vi "simple_tsv_recording.vi"(7 "file_base_name":string="simple_record", 8 "value":dbl format="%#_13g", 11 "date_time":timestamp) -> ()   [LabVIEW 2019]
uses:
  <vilib>/Utility/file.llb/Write Delimited Spreadsheet (string).vi
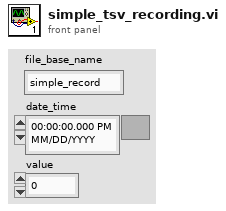
[diagram p1: front panel]
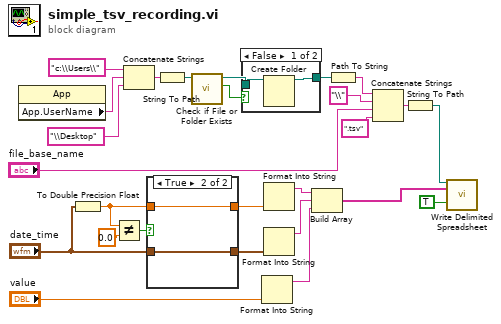
[diagram p0: block diagram]
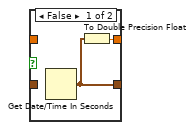
[diagram p2: hidden frame]
diagram:
  n1 = property class="App"() -> ("App.UserName"=w23:string)  [unwired: 2 in, 2 out]
  n2 = To Double Precision Float(number="date_time") -> (double precision float=w1:dbl)
  n3 = Not Equal?(x=w1, y=0.0) -> (x != y?=w9:bool)
  n4 = Concatenate Strings("c:\\Users\\", w23, "\\Desktop") -> (w21:string)
  n5 = case shown="True" w9 {
    tunnel: [w27 w30] -> w6
    tunnel: "date_time" -> [_ w30]
    tunnel: [w28 w29] -> w2
    tunnel: w1 -> [_ w29]
    frame False {
      n6 = Get Date/Time In Seconds() -> (seconds since 1Jan1904=w27:timestamp)
      n7 = To Double Precision Float(number=w27) -> (double precision float=w28:dbl)
    }
    frame True {
    }
  }
  n8 = String To Path(string=w21) -> (path=w16:path)
  n9 = call <vilib>:"Check if File or Folder Exists.vi"("path"=w16) -> ("file or folder exists?"=w15:bool, "dup path"=w13:path)  [unwired: 8 in, 1 out]
  n10 = case shown="False" w15 {
    tunnel: w13 -> [w32 w33]
    tunnel: [w31 w33] -> w14
    frame False {
      n11 = Create Folder(path (use dialog)=w32) -> (created path=w31:path)  [unwired: 2 in, 2 out]
    }
    frame True {
    }
  }
  n12 = Format Into String("value") -> (resulting string=w3:string)  [unwired: 3 in, 1 out]
  n13 = Format Into String(w2) -> (resulting string=w5:string)  [unwired: 3 in, 1 out]
  n14 = Format Into String(w6) -> (resulting string=w4:string)  [unwired: 3 in, 1 out]
  n15 = Build Array(w5, w4, w3) -> (w26:string[])
  n16 = Path To String(path=w14) -> (string=w12:string)
  n17 = Concatenate Strings(w12, "\\", "file_base_name", ".tsv" ("string")) -> (w17:string)
  n18 = String To Path(string=w17) -> (path=w11:path)
  n19 = call-poly <vilib>:"Write Delimited Spreadsheet.vi"("file path (dialog if empty)"=w11, "1D data"=w26, "append to file? (new file:F)"=TRUE) -> ()  [unwired: 11 in, 2 out]
